vi "AgreedClassLayerDeserialize.vi"(7 "ClassOp":T1={"Layer"=enum."new class layer", "SerializedClassName"="", "default data?"=FALSE, "BlueSerializableVersion"={"From"=0, "To"=0}, "object"={"default object"=refnum, "SerializableDataOverride"=variant(cluster{"SerializableData":variant, "Use?":bool} {"SerializableData"=variant, "Use?"=FALSE}), "UseSerializableDataOverride?"=FALSE}}, 8 "error in (no error)":errorcluster, 9 "SerializableData":variant, 10 "StructuredData":variant, 11 "BlueSerializer in":refnum<class "BlueSerializer.lvclass">) -> (0 "error out":errorcluster, 1 "Variant":variant, 2 "StructuredData":variant, 3 "BlueSerializer out":refnum<class "BlueSerializer.lvclass">)   [LabVIEW 2020, in "BlueSerialization.lvlib" / "BlueSerializer.lvclass"]
uses:
  BlueSerializer.lvclass
  Support/SetSerializableDataClusterIterable.ctl
  BlueSerializable/BlueSerializable.lvclass
  Support/SetSerializableDataClusterLayer.ctl
  BlueSerializableVersion.ctl
  Support/SetSerializableDataObject.ctl
  <vilib>/Utility/error.llb/Error Cluster From Error Code.vi
  <vilib>/ErrorRing/Error Ring.xnode
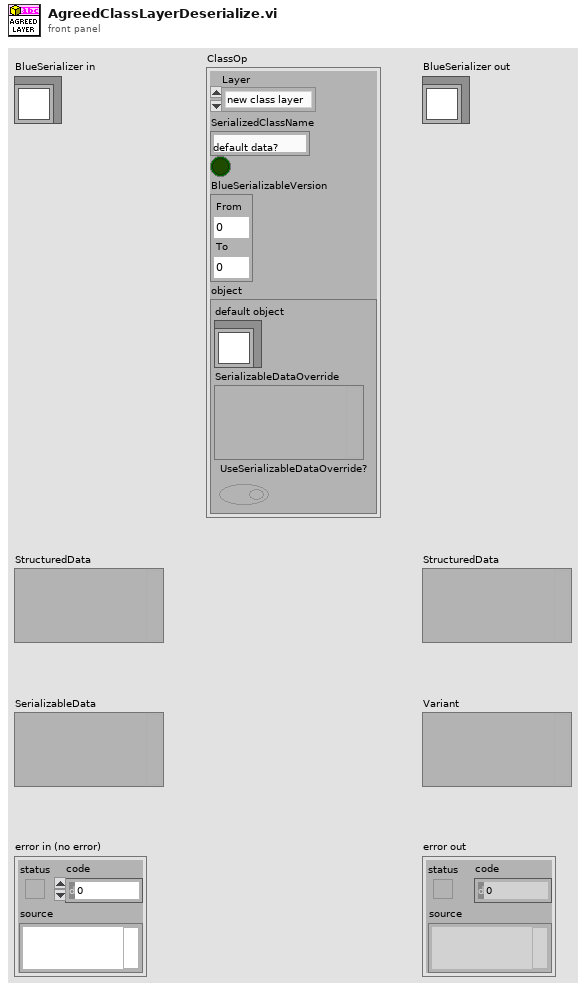
[diagram p1: front panel]
types:
  T1 = typedef "BlueSerialization.lvlib/BlueSerializer.lvclass/SetSerializableDataClusterIterable.ctl" = cluster{"Layer":T2, "SerializedClassName":string, "default data?":bool, "BlueSerializableVersion":T3, "object":T4}
  T2 = typedef "BlueSerialization.lvlib/BlueSerializer.lvclass/SetSerializableDataClusterLayer.ctl" = enum16{"new class layer", "dropped class layer", "agreed class layer"}
  T3 = typedef "BlueSerialization.lvlib/BlueSerializer.lvclass/BlueSerializableVersion.ctl" = cluster{"From":u16, "To":u16}
  T4 = typedef "BlueSerialization.lvlib/BlueSerializer.lvclass/SetSerializableDataObject.ctl" = cluster{"default object":refnum<class "BlueSerializable.lvclass">, "SerializableDataOverride":variant, "UseSerializableDataOverride?":bool}
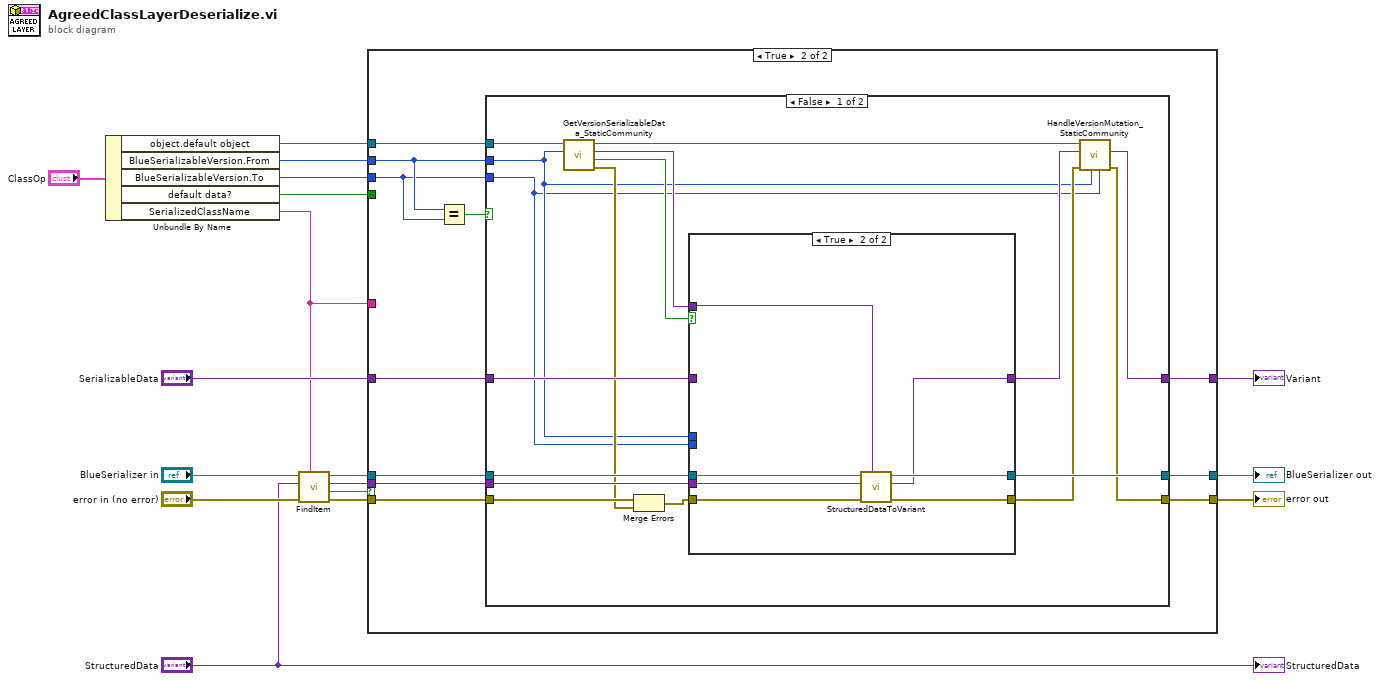
[diagram p0: block diagram]
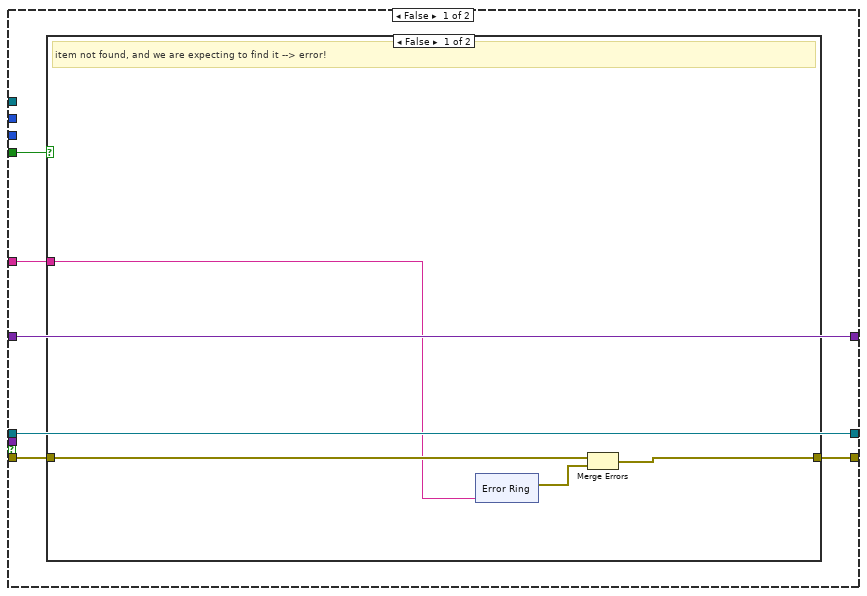
[diagram p2: hidden frame]
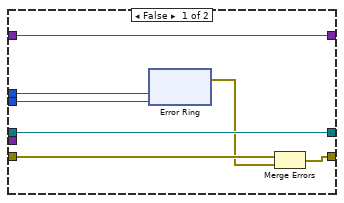
[diagram p4: hidden frame]
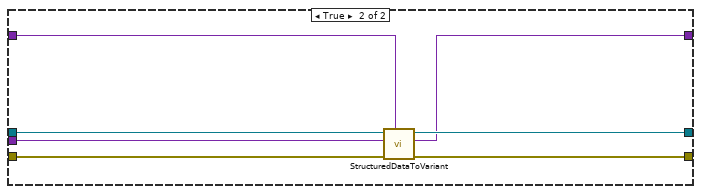
[diagram p5: hidden frame]
diagram:
  n1 = Unbundle By Name("ClassOp") -> ("object.default object"=w6:refnum<class "BlueSerializable.lvclass">, "BlueSerializableVersion.From"=w4:u16, "BlueSerializableVersion.To"=w3:u16, "default data?"=w1:bool, "SerializedClassName"=w7:string)
  n2 = call-dynamic "FindItem.vi"("Item Name"=w7, "error in (no error)"="error in (no error)", "StructuredDataContainer"="StructuredData", "BlueSerializer in"="BlueSerializer in") -> ("error out"=w12:errorcluster, "Found?"=w11:bool, "StructuredDataItem"=w17:variant, "BlueSerializer out"=w13:refnum<class "BlueSerializer.lvclass">)  [unwired: 4 in]
  n3 = case shown="True" w11 {
    tunnel: w13 -> [w20 w38]
    tunnel: w12 -> [w22 w36]
    tunnel: "SerializableData" -> [w23 w39]
    tunnel: [w20 w46] -> w15
    tunnel: [w23 w45] -> w16
    tunnel: [w21 w44] -> w14
    tunnel: w17 -> [_ w37]
    tunnel: w7 -> [w19 _]
    tunnel: w6 -> [_ w43]
    tunnel: w4 -> [_ w41]
    tunnel: w3 -> [_ w40]
    tunnel: w1 -> [w18 _]
    frame False {
      n4 = case shown="False" w18 {
        tunnel: w22 -> [w27 w35]
        tunnel: [w26 w35] -> w21
        tunnel: w19 -> [w24 _]
        frame False {
          # "item not found, and we are expecting to find it --> error!"
          n5 = xnode "Error Ring"("parameter 0"=w24) -> ("error out"=w25:errorcluster)
          n6 = Merge Errors(w27, w25) -> (w26:errorcluster)
        }
        frame True {
          # "Don't error if we find the default data flag in the header"
        }
      }
    }
    frame True {
      n7 = Equal?(x=w41, y=w40) -> (x = y?=w42:bool)
      n8 = case shown="False" w42 {
        tunnel: [w63 w92] -> w46
        tunnel: [w51 w91] -> w45
        tunnel: [w47 w90] -> w44
        tunnel: w37 -> [w62 w89]
        tunnel: w38 -> [w61 w88]
        tunnel: w39 -> [w60 w87]
        tunnel: w36 -> [w59 w86]
        tunnel: w43 -> [w57 _]
        tunnel: w41 -> [w49 _]
        tunnel: w40 -> [w48 _]
        frame False {
          n9 = call "GetVersionSerializableData_StaticCommunity.vi"("Version"=w49, "BlueSerializable in"=w57) -> ("error out"=w54:errorcluster, "Found?"=w55:bool, "SerializableData"=w56:variant, "BlueSerializable out"=w53:refnum<class "BlueSerializable.lvclass">)  [unwired: 6 in]
          n10 = Merge Errors(w59, w54) -> (w58:errorcluster)
          n11 = case shown="True" w55 {
            tunnel: [w69 w85] -> w63
            tunnel: [w70 w84] -> w52
            tunnel: [w67 w83] -> w50
            tunnel: w62 -> [_ w82]
            tunnel: w61 -> [w69 w81]
            tunnel: w60 -> [w70 _]
            tunnel: w58 -> [w68 w80]
            tunnel: w49 -> [w66 _]
            tunnel: w48 -> [w65 _]
            tunnel: w56 -> [_ w79]
            frame False {
              n12 = xnode "Error Ring"("parameter 0"=w66, "parameter 1"=w65) -> ("error out"=w64:errorcluster)
              n13 = Merge Errors(w68, w64) -> (w67:errorcluster)
            }
            frame True {
              n14 = call-dynamic "StructuredDataToVariant.vi"("Data Type"=w79, "error in (no error)"=w80, "StructuredData"=w82, "BlueSerializer in"=w81) -> ("error out"=w83:errorcluster, "Variant"=w84:variant, "BlueSerializer out"=w85:refnum<class "BlueSerializer.lvclass">)  [unwired: 5 in]
            }
          }
          n15 = call "HandleVersionMutation_StaticCommunity.vi"("To Version"=w48, "From Version"=w49, "error in (no error)"=w50, "SerializableData in"=w52, "BlueSerializable in"=w53) -> ("error out"=w47:errorcluster, "SerializableData out"=w51:variant)  [unwired: 4 in, 1 out]
        }
        frame True {
          n16 = call-dynamic "StructuredDataToVariant.vi"("Data Type"=w87, "error in (no error)"=w86, "StructuredData"=w89, "BlueSerializer in"=w88) -> ("error out"=w90:errorcluster, "Variant"=w91:variant, "BlueSerializer out"=w92:refnum<class "BlueSerializer.lvclass">)  [unwired: 5 in]
        }
      }
    }
  }
  "error out" <- w14
  "BlueSerializer out" <- w15
  "Variant" <- w16
  "StructuredData" <- "StructuredData"
